vi "notificacoes.vi"(11 "String":string) -> (3 "This VI":refnum<vi>)   [LabVIEW 2018]
panel:
  out "Atenção":string
  in  "Fechar":bool
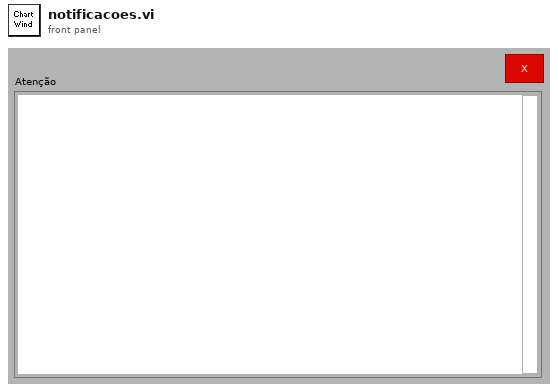
[diagram p1: front panel]
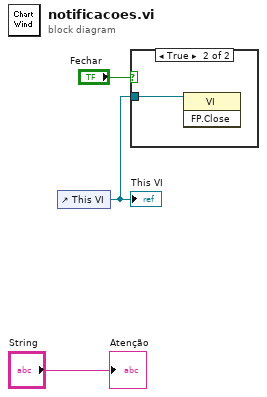
[diagram p0: block diagram]
diagram:
  n1 = control-ref of="This VI"() -> (w3:refnum<vi>)
  "This VI" <- w3
  n2 = case shown="True" "Fechar" {
    tunnel: w3 -> [_ w4]
    frame False {
    }
    frame True {
      n3 = invoke class="VI" method="FP.Close"(reference=w4) -> ()  [unwired: 2 in, 3 out]
    }
  }
  "Atenção" <- "String"
